vi "Main3.vi"() -> ()   [LabVIEW 2014]
doc: "The myRIO Project template acquires acceleration data from the onboard accelerometer and displays the changes of acceleration values in a waveform chart."
uses:
  C:/Program Files (x86)/National Instruments/LabVIEW 2014/examples/robotics/Vision/Color Tracking/HueSlider.ctl
  <vilib>/myRIO/Instrument Drivers/Onboard IO/AI/typedefs/AI Reference.ctl
  <vilib>/myRIO/Common/Instrument Driver Framework/Utilities/typedefs/myRIO Generic Hardware Reference.ctl
  <vilib>/myRIO/Common/Instrument Driver Framework/Utilities/typedefs/Hardware Version Enum.ctl
  <vilib>/myRIO/Common/Instrument Driver Framework/Utilities/typedefs/myRIO v1.0 Reference.ctl
  <vilib>/myRIO/Common/Instrument Driver Framework/Utilities/typedefs/Generic FPGA Reference.ctl
  <vilib>/myRIO/Common/Instrument Driver Framework/myRIO v1.0/AI/typedefs/AI Channels List.ctl
  <vilib>/myRIO/Common/Instrument Driver Framework/myRIO v1.0/AI/typedefs/AI Channels Enum.ctl
  <vilib>/myRIO/Common/Instrument Driver Framework/Utilities/typedefs/Analog Scaling Constants List.ctl
  <vilib>/myRIO/Common/Instrument Driver Framework/Utilities/typedefs/Analog Scaling Constants.ctl
  <vilib>/userdefined/High Color/nirio_resource_hc.ctl
  <vilib>/myRIO/Instrument Drivers/Onboard IO/PWM/typedefs/PWM Reference.ctl
  <vilib>/myRIO/Common/Instrument Driver Framework/myRIO v1.0/PWM/typedefs/PWM Channels Enum.ctl
  <vilib>/myRIO/Instrument Drivers/Onboard IO/PWM/typedefs/PWM Configuration.ctl
  <vilib>/myRIO/Common/Instrument Driver Framework/Utilities/vis/Is FPGA Ref Available.vi
  <vilib>/myRIO/Common/Instrument Driver Framework/myRIO v1.0/AI/vis/myRIO v1.1 Open AI.vi
  <vilib>/myRIO/Instrument Drivers/Onboard IO/AI/vis/Read.vi
  <vilib>/myRIO/Common/Instrument Driver Framework/myRIO v1.0/PWM/vis/myRIO v1.1 Open PWM.vi
  <vilib>/myRIO/Instrument Drivers/Onboard IO/PWM/vis/Set Duty Cycle and Frequency.vi
  <vilib>/myRIO/Common/Instrument Driver Framework/Utilities/vis/Validate Channels.vi
  <vilib>/myRIO/Common/Instrument Driver Framework/myRIO v1.0/AI/vis/myRIO v1.0 Reserve AI.vi
  <vilib>/myRIO/Common/Instrument Driver Framework/myRIO v1.0/PWM/vis/myRIO v1.0 Reserve PWM.vi
  <vilib>/myRIO/Common/Instrument Driver Framework/myRIO v1.0/AI/vis/myRIO v1.0 Build MUX Configuration AI.vi
  <vilib>/myRIO/Common/Instrument Driver Framework/myRIO v1.0/Resource Manager/vis/myRIO v1.0 Reserve Channel List.vi
  <vilib>/myRIO/Common/Instrument Driver Framework/myRIO v1.0/PWM/vis/myRIO v1.0 Build MUX Configuration PWM.vi
  <vilib>/myRIO/Common/Instrument Driver Framework/myRIO v1.0/Resource Manager/vis/myRIO v1.0 Reserve Channel.vi
  <vilib>/myRIO/Common/Instrument Driver Framework/myRIO v1.0/Resource Manager/vis/myRIO v1.0 Unreserve Channel.vi
  <vilib>/myRIO/Common/Instrument Driver Framework/myRIO v1.0/Resource Manager/vis/myRIO v1.0 Create Configuration List.vi
  <vilib>/myRIO/Common/Instrument Driver Framework/myRIO v1.0/Resource Manager/vis/myRIO v1.0 Build Mutex Name.vi
  <vilib>/Utility/VariantDataType/GetNumericInfo.vi
  <vilib>/Utility/error.llb/Error Cluster From Error Code.vi
  <vilib>/myRIO/Common/Instrument Driver Framework/myRIO v1.0/myRIO v1.1 Open.vi
  <vilib>/myRIO/Common/Instrument Driver Framework/myRIO v1.0/AI/vis/myRIO v1.0 Get Scaling Constants AI.vi
  <vilib>/myRIO/Common/Instrument Driver Framework/Utilities/vis/IO Manager.vi
  <vilib>/myRIO/Common/Instrument Driver Framework/Utilities/vis/Configuration Manager.vi
  <vilib>/myRIO/Common/Instrument Driver Framework/myRIO v1.0/myRIO v1.0 Close.vi
  <vilib>/myRIO/Common/Instrument Driver Framework/myRIO v1.0/AI/vis/myRIO v1.0 Read AI.vi
  <vilib>/myRIO/Common/Instrument Driver Framework/myRIO v1.0/Resource Manager/vis/myRIO v1.0 Configure IO.vi
  <vilib>/myRIO/Common/Instrument Driver Framework/myRIO v1.0/PWM/vis/myRIO v1.0 Write PWM.vi
  <vilib>/myRIO/Express VI/Onboard IO/AI/AI Express VI.xnode
  <vilib>/myRIO/Instrument Drivers/Onboard IO/AI/vis/myRIO AI Open.xnode
  <vilib>/myRIO/Express VI/Onboard IO/PWM/PWM Express VI.xnode
  <vilib>/myRIO/Instrument Drivers/Onboard IO/PWM/vis/myRIO PWM Open.xnode
  <vilib>/myRIO/Instrument Drivers/Onboard IO/PWM/PWM.lvlib
  <vilib>/vision/driver/NI_Vision_Acquisition_Software.lvlib
  <vilib>/vision/NI_Vision_Development_Module.lvlib
  <vilib>/myRIO/Instrument Drivers/Onboard IO/AI/AI.lvlib
panel:
  out "웨이브폼 차트":dbl(graph)
  out "Image 2":T1(plugin-control)
  in  "Hue range":T2={"Min"=232, "Max"=21} scale=0.0..255.0
  in  "Stop 2":bool
  out "Image":T1(plugin-control)
  in  "Camera Name":refnum<k21>="cam3" caption="IMAQdx Session"
  # "Control Motor"
  # "Read Encoder"
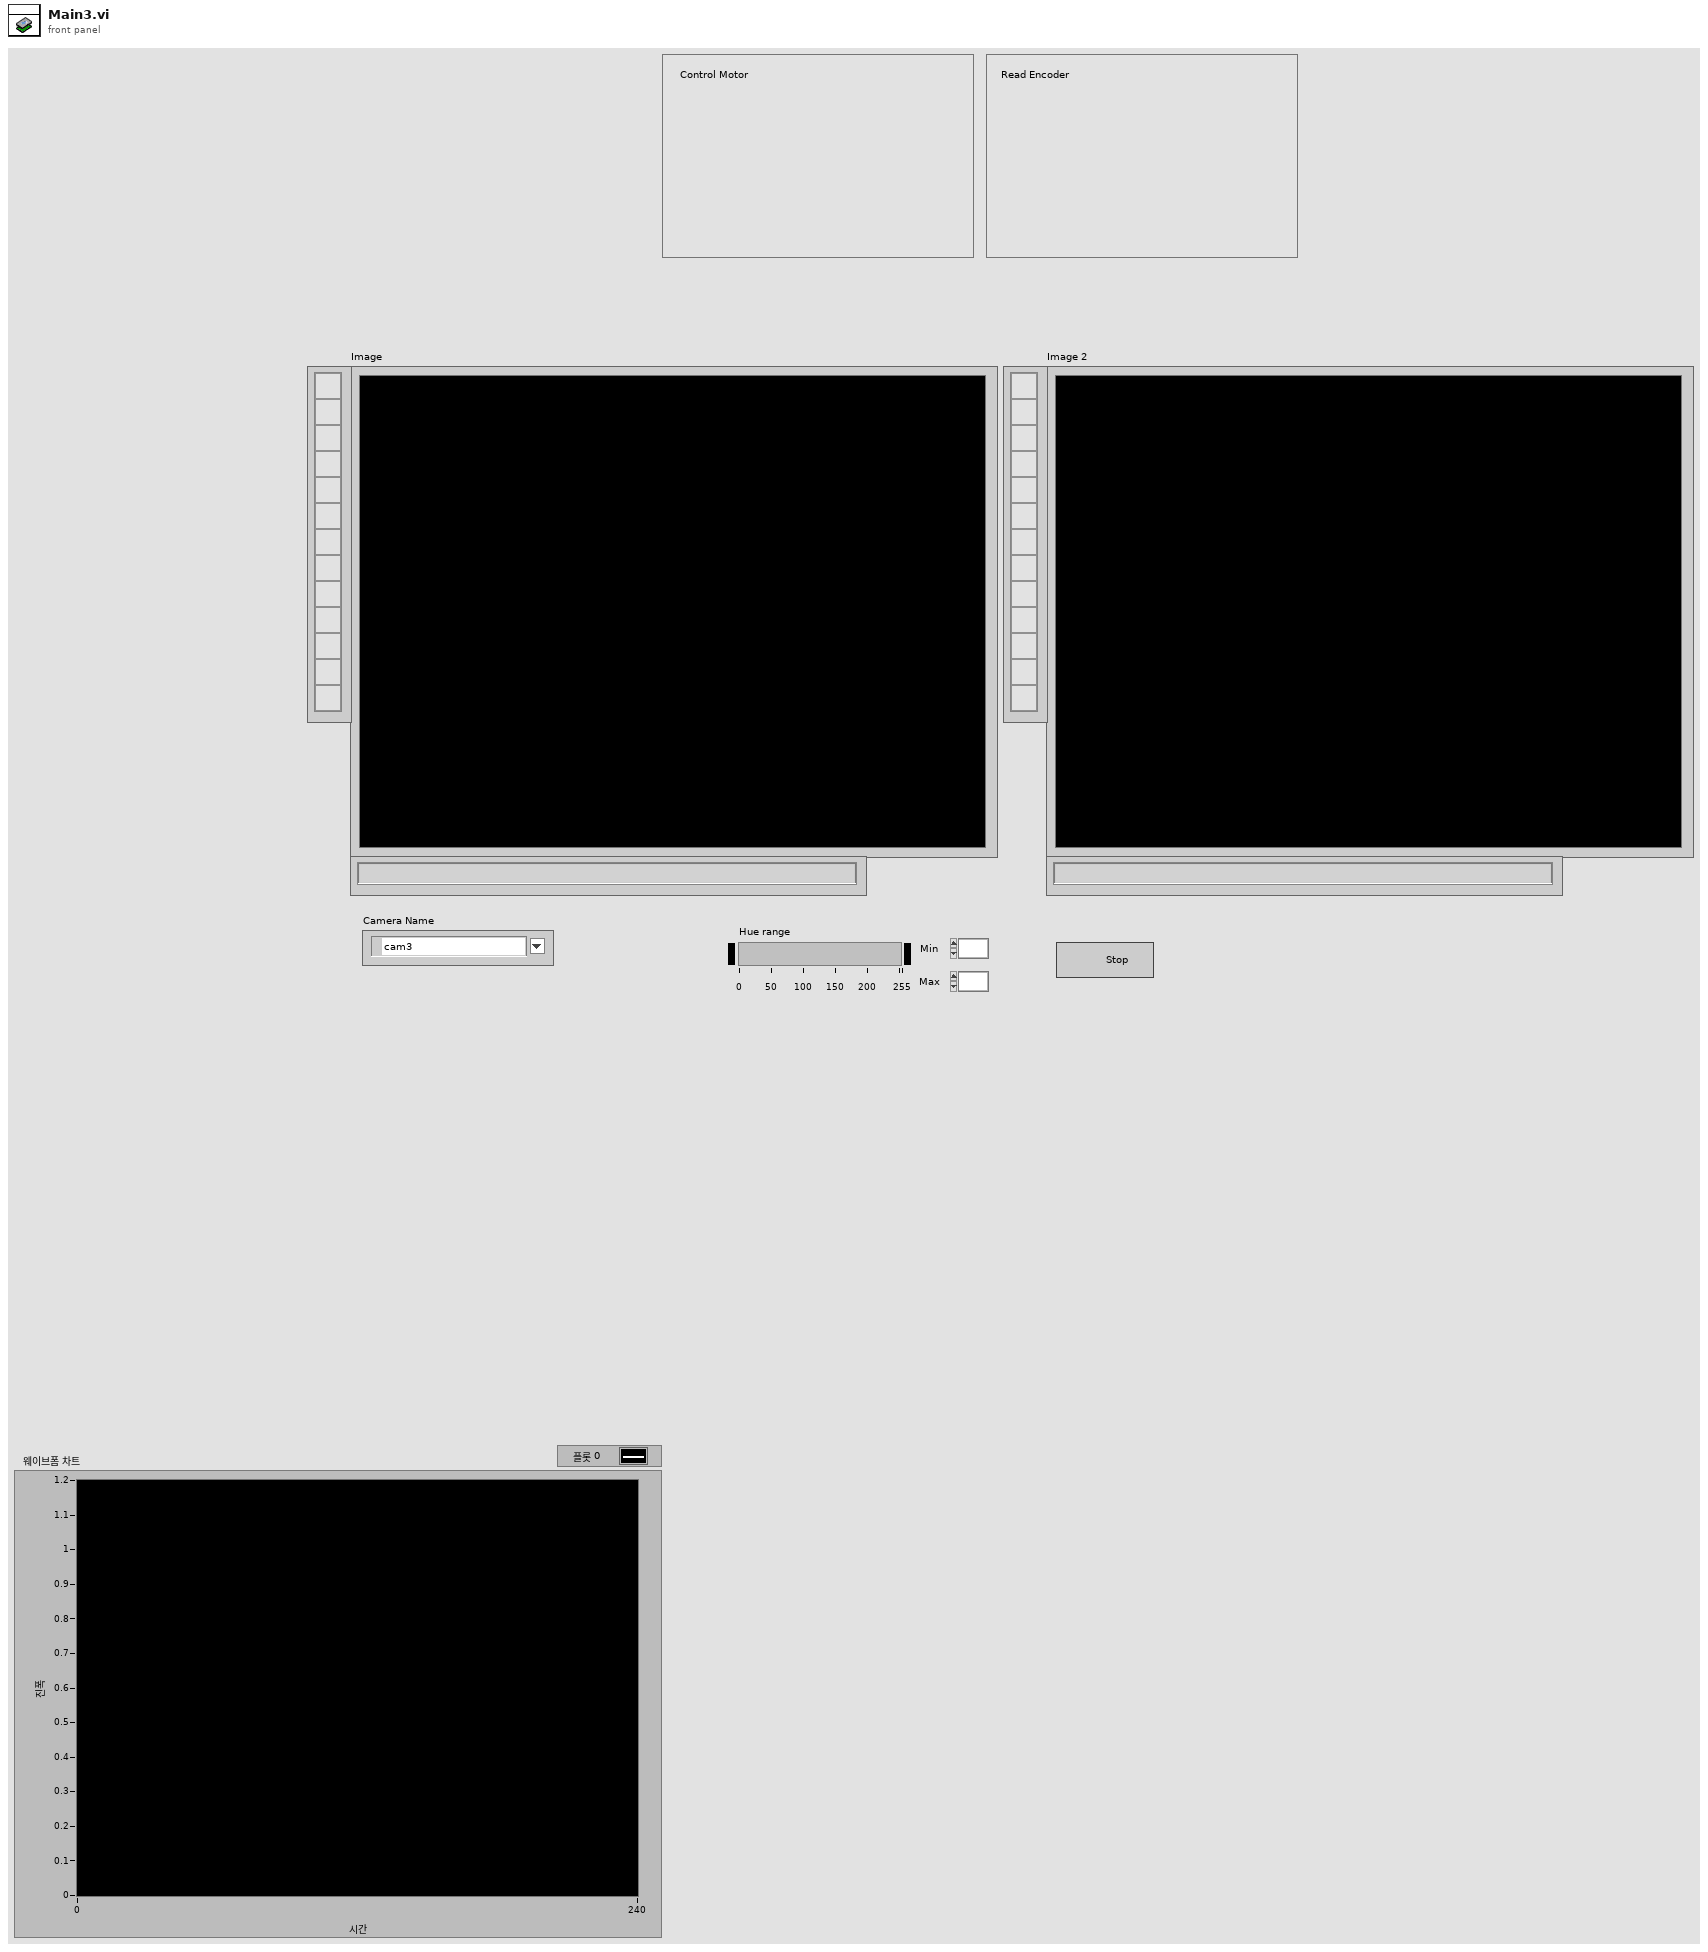
[diagram p1: front panel]
types:
  T1 = typedef "IMAQ Image.ctl" = refnum<image>
  T2 = typedef "HueSlider.ctl" = cluster{"Min":i32, "Max":i32}
  T3 = typedef "IMAQ Circle" = cluster{"Center X":i32, "Center Y":i32, "Inner Radius":i32, "Outer Radius":i32, "Start Angle":dbl, "End Angle":dbl}
  T4 = typedef "AI.lvlib/AI Reference.ctl" = cluster{"myRIO Reference":T5, "AI Channels List":T9, "AI Scaling Constants List":T11}
  T5 = typedef "myRIO Generic Hardware Reference.ctl" = cluster{"myRIO Model":T6, "myRIO Hardware Reference":T7}
  T6 = typedef "Hardware Version Enum.ctl" = enum16{"Unknown", "myRIO-1900", "myRIO-1950"}
  T7 = typedef "myRIO v1.0 Reference.ctl" = cluster{"Generic FPGA Reference":T8, "Allow multiple opens":bool}
  T8 = typedef "Generic FPGA Reference.ctl" = refnum<k20>
  T9 = typedef "AI Channels List.ctl" = T10[]
  T10 = typedef "AI Channels Enum.ctl" = enum16{"Not Connected", "AudioIn/Left", "AudioIn/Right", "C/AI0", "C/AI1", "A/AI0", "A/AI1", "A/AI2", "A/AI3", "B/AI0", "B/AI1", "B/AI2", "B/AI3"}
  T11 = typedef "Analog Scaling Constants List.ctl" = T12[]
  T12 = typedef "Analog Scaling Constants.ctl" = cluster{"LSB Weight (Volts)":dbl, "Offset (Volts)":dbl, "Signed?":bool}
  T13 = typedef "nirio_resource_hc.ctl" = tag
  T14 = typedef "IMAQ Rectangle" = cluster{"Left":i32, "Top":i32, "Right":i32, "Bottom":i32, "Rotation":dbl}
  T15 = typedef "PWM.lvlib/PWM Reference.ctl" = cluster{"myRIO Reference":T5, "PWM Channels Enum":T16, "PWM Configuration":T17}
  T16 = typedef "PWM Channels Enum.ctl" = enum16{"Not Connected", "C/PWM0", "C/PWM1", "A/PWM0", "A/PWM1", "A/PWM2", "B/PWM0", "B/PWM1", "B/PWM2"}
  T17 = typedef "PWM.lvlib/PWM Configuration.ctl" = cluster{"Frequency":dbl, "Duty Cycle":dbl}
  T18 = typedef "IMAQdx.ctl" = refnum<k21>
  T19 = cluster{"Global Rectangle":i32[], "Contours":cluster{"Contour Type":u32, "ROI Type":u32, "Points":i32[]}[]}
  T20 = cluster{"Center":cluster{"X":sgl, "Y":sgl}, "Radius":dbl}
  T21 = typedef "ROI Descriptor" = cluster{"Global Rectangle":i32[], "Contours":cluster{"ID":enum32{"External", "Internal"}, "Type":u32, "Coordinates":i32[]}[]}
  T22 = cluster{"Area":dbl, "Number of Holes":dbl, "Bounding Rect":cluster{"Left":dbl, "Top":dbl, "Right":dbl, "Bottom":dbl}, "Center of Mass":cluster{"X":dbl, "Y":dbl}, "Orientation":dbl, "Dimensions":cluster{"Width":dbl, "Height":dbl}}[]
  T23 = cluster{"Left":dbl, "Top":dbl, "Right":dbl, "Bottom":dbl}
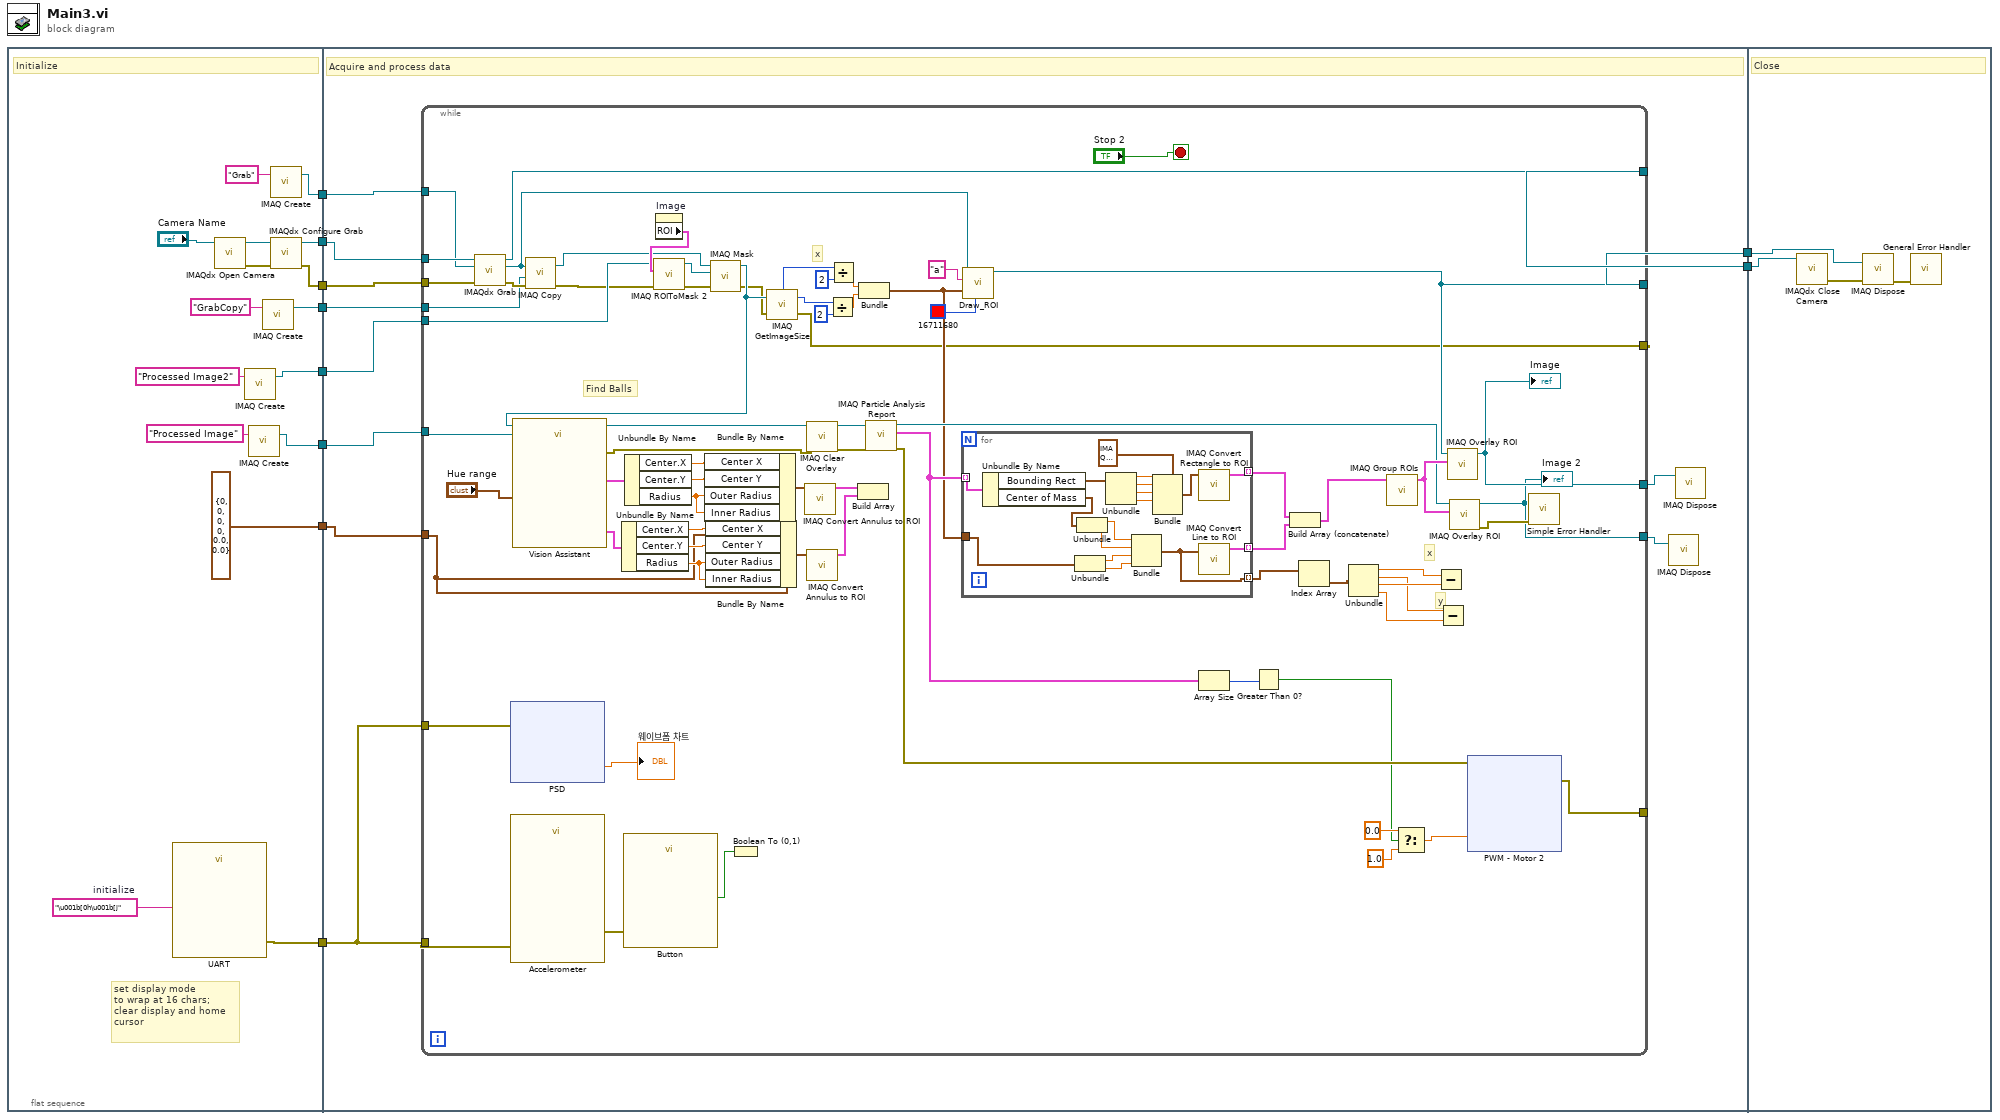
[diagram p0: block diagram]
diagram:
  n1 = flat-sequence {
    tunnel: [w22] -> w10
    tunnel: [w21] -> w9
    tunnel: [w20] -> w8
    tunnel: [T3 {"Center X"=0, "Center Y"=0, "Inner Radius"=0, "Outer Radius"=0, "Start Angle"=0.0, "End Angle"=0.0} ("Annulus")] -> w5
    tunnel: [w17] -> w4
    tunnel: [w15] -> w3
    tunnel: [w13] -> w2
    tunnel: [w12] -> w1
    tunnel: w10 -> [w38]
    tunnel: w9 -> [w37]
    tunnel: w8 -> [w36]
    tunnel: [w28] -> w7
    tunnel: [w35] -> w6
    tunnel: w5 -> [w34]
    tunnel: w4 -> [w33]
    tunnel: w3 -> [w30]
    tunnel: w2 -> [w29]
    tunnel: w1 -> [w27]
    tunnel: w7 -> [w202]
    tunnel: w6 -> [w201]
    frame #0 {
      w11 = "\u001b[0h\u001b[j"  # initialize
      # "set display mode\nto wrap at 16 chars;\nclear display and home\ncursor"
      # "Initialize"
      n2 = call "UART"("Characters to Write"=w11) -> ("error out"=w12:errorcluster)  [unwired: 25 in, 1 out]
      n3 = call <vilib>:"IMAQdx Open Camera.vi"("Session In"="Camera Name") -> ("error out"=w26:errorcluster, "Session Out"=w25:T18)  [unwired: 2 in, 7 out]
      n4 = call "IMAQ Create"("Image Name"="Processed Image2") -> ("New Image"=w15:T1)  [unwired: 3 in, 2 out]
      n5 = call "IMAQ Create"("Image Name"="Processed Image") -> ("New Image"=w17:T1)  [unwired: 3 in, 2 out]
      n6 = call "IMAQ Create"("Image Name"="GrabCopy") -> ("New Image"=w13:T1)  [unwired: 3 in, 2 out]
      n7 = call "IMAQ Create"("Image Name"="Grab") -> ("New Image"=w22:T1)  [unwired: 3 in, 2 out]
      n8 = call <vilib>:"IMAQdx Configure Grab.vi"("error in"=w26, "Session In"=w25) -> ("error out"=w20:errorcluster, "Session Out"=w21:T18)  [unwired: 8 out]
    }
    frame #1 {
      # "Acquire and process data"
      n9 = while {
        tunnel: [w108] -> w35
        tunnel: w36 -> [w110]
        tunnel: w37 -> [w111]
        tunnel: w38 -> [w109]
        tunnel: w34 -> [w90]
        tunnel: w33 -> [w89]
        tunnel: [w88] -> _
        tunnel: [w55] -> w32
        tunnel: [w54] -> w31
        tunnel: w30 -> [w78]
        tunnel: w29 -> [w63]
        tunnel: [w56] -> w28
        tunnel: [w52] -> _
        tunnel: w27 -> [w49]
        tunnel: w27 -> [w40]
        stop <- "Stop 2" stop-if-true
        # "y"
        # "x"
        # "x"
        # "Find Balls"
        n10 = call <vilib>:"IMAQdx Grab.vi"("error in"=w110, "Image In"=w109, "Session In"=w111) -> ("error out"=w65:errorcluster, "Image Out"=w61:T1, "Session Out"=w108:T18)  [unwired: 1 in, 5 out]
        n11 = xnode "PSD"("error in (no error)"=w40) -> ("C/AI0 (C/AI0 (AI0))"=→"웨이브폼 차트":dbl)  [unwired: 1 out]
        n12 = call "Accelerometer"("error in (no error)"=w49) -> ("error out"=w50:errorcluster)  [unwired: 23 in, 3 out]
        n13 = call "IMAQ Copy"("error in (no error)"=w65, "Image Dst"=w63, "Image Src"=w61) -> ("error out"=w64:errorcluster, "Image Dst Out"=w62:T1)  [unwired: 3 in]
        n14 = call "Button"("error in (no error)"=w50) -> ("Value"=w51:bool)  [unwired: 25 in, 1 out]
        n15 = property on="Image" class="ImageControl"() -> ("ROI"=w80:T19)  [unwired: 2 in, 2 out]
        n16 = call "IMAQ ROIToMask 2"("error in (no error)"=w64, "ROI Descriptor"=w80, "Image"=w78) -> ("error out"=w76:errorcluster, "Image Out"=w77:T1)  [unwired: 6 in, 1 out]
        n17 = call "IMAQ Mask"("error in (no error)"=w76, "Image Mask"=w77, "Image Src"=w62) -> ("error out"=w53:errorcluster, "Image Dst Out"=w60:T1)  [unwired: 2 in]
        n18 = call "Vision Assistant"("Image In"=w60, "Image Dst"=w89, "Red or Hue Range (Color Threshold)"="Hue range") -> ("Image Out"=w103:T1, "Best Circle (Fit Circle Ball 1)"=w91:T20, "Best Circle (Fit Circle Ball 2)"=w100:T20, "error out"=w105:errorcluster)  [unwired: 1 in, 20 out]
        n19 = Unbundle By Name(w100) -> ("Center.X"=w94:sgl, "Center.Y"=w95:sgl, "Radius"=w101:dbl)
        n20 = Unbundle By Name(w91) -> ("Center.X"=w92:sgl, "Center.Y"=w93:sgl, "Radius"=w102:dbl)
        n21 = Bundle By Name(cluster=w90, "Center X"=w92, "Center Y"=w93, "Outer Radius"=w102, "Inner Radius"=w102) -> (w96:T3)
        n22 = Bundle By Name(cluster=w90, "Center X"=w94, "Center Y"=w95, "Outer Radius"=w101, "Inner Radius"=w101) -> (w97:T3)
        n23 = Boolean To (0,1)(Boolean=w51) -> ()  [unwired: 1 out]
        n24 = call "IMAQ GetImageSize"("Image"=w60, "error in (no error)"=w53) -> ("Y Resolution"=w70:i32, "X Resolution"=w73:i32, "error out"=w52:errorcluster)  [unwired: 2 in]
        n25 = call "IMAQ Convert Annulus to ROI"("Annulus"=w96) -> ("ROI Descriptor"=w98:T21)  [unwired: 1 in, 8 out]
        n26 = call "IMAQ Clear Overlay"("error in (no error)"=w105, "Image"=w103) -> ("error out"=w74:errorcluster, "Image Out"=w83:T1)  [unwired: 1 in, 7 out]
        n27 = call "IMAQ Convert Annulus to ROI"("Annulus"=w97) -> ("ROI Descriptor"=w99:T21)  [unwired: 1 in, 8 out]
        n28 = Divide(x=w70, y=2) -> (x/y=w68:dbl)
        n29 = Divide(x=w73, y=2) -> (x/y=w69:dbl)
        n30 = Build Array(w98, w99) -> ()  [unwired: 1 out]
        n31 = Bundle(w69, w68) -> (w59:cluster{dbl, dbl})  [unwired: 1 in]
        n32 = call "IMAQ Particle Analysis Report"("error in (no error)"=w74, "Image"=w83) -> ("error out"=w81:errorcluster, "Particle Reports (Pixels)"=w75:T22, "Image Out (duplicate)"=w82:T1)  [unwired: 4 in, 3 out]
        n33 = for {
          tunnel: w75 -> [w165] mode=indexing
          tunnel: [w157] -> w58 mode=indexing
          tunnel: w59 -> [w153]
          tunnel: [w150] -> w48 mode=indexing
          tunnel: [w149] -> w47 mode=indexing
          n34 = Unbundle By Name(w165) -> ("Bounding Rect"=w163:T23, "Center of Mass"=w156:cluster{"X":dbl, "Y":dbl})
          n35 = Unbundle(w153) -> (w152:dbl, w151:dbl)
          n36 = Unbundle(w156) -> ("X"=w155:dbl, "Y"=w154:dbl)
          n37 = Unbundle(w163) -> ("Left"=w162:dbl, "Top"=w161:dbl, "Right"=w160:dbl, "Bottom"=w159:dbl)
          n38 = Bundle("X"=w155, "Y"=w154, w152, w151) -> (w149:cluster{"X":dbl, "Y":dbl, dbl, dbl})  [unwired: 1 in]
          n39 = Bundle(cluster=T14 {"Left"=0, "Top"=0, "Right"=0, "Bottom"=0, "Rotation"=0.0} ("Rectangle"), "Left"=w162, "Top"=w161, "Right"=w160, "Bottom"=w159) -> (w158:T14)  [unwired: 1 in]
          n40 = call "IMAQ Convert Rectangle to ROI"("Rectangle"=w158) -> ("ROI Descriptor"=w157:T21)  [unwired: 8 in, 1 out]
          n41 = call "IMAQ Convert Line to ROI"("Line"=w149) -> ("ROI Descriptor"=w150:T21)  [unwired: 8 in, 1 out]
        }
        n42 = call "Draw_ROI.vi"("Color"=u32 16711680, "클러스터"=w59, "Group"="a", "참조 번호 입력"=w61) -> ("참조 번호 출력"=w56:T1)  [unwired: 7 in]
        n43 = Array Size(array=w75) -> (size(s)=w87:i32)
        n44 = Greater Than 0?(x=w87) -> (x > 0?=w39:bool)
        n45 = Build Array (concatenate)(w58, w48) -> (w57:T21[])
        n46 = Index Array(array=w47) -> (element=w46:cluster{"X":dbl, "Y":dbl, dbl, dbl})  [unwired: 1 in]
        n47 = Unbundle(w46) -> ("X"=w45:dbl, "Y"=w43:dbl, w44:dbl, w42:dbl)
        n48 = call "IMAQ Group ROIs"("ROI Descriptors"=w57) -> ("ROI Descriptor out"=w104:T21)  [unwired: 1 in, 3 out]
        n49 = Select(t=0.0, s=w39, f=1.0) -> (s? t:f=w84:dbl)
        n50 = Subtract(x=w45, y=w44) -> ()  [unwired: 1 out]
        n51 = Subtract(x=w43, y=w42) -> ()  [unwired: 1 out]
        n52 = call "IMAQ Overlay ROI"("ROI Descriptor"=w104, "Image"=w56) -> ("Image Out"=w55:T1)  [unwired: 4 in, 5 out]
        "Image" <- w55
        n53 = call "IMAQ Overlay ROI"("ROI Descriptor"=w104, "Image"=w82) -> ("error out"=w106:errorcluster, "Image Out"=w54:T1)  [unwired: 4 in, 4 out]
        "Image 2" <- w54
        n54 = xnode "PWM - Motor 2"("Duty Cycle"=w84, "error in (no error)"=w81) -> ("error out"=w88:errorcluster)
        n55 = call <vilib>:"Simple Error Handler.vi"("error in (no error)"=w106) -> ()  [unwired: 1 in, 8 out]
      }
      n56 = call "IMAQ Dispose"("Image"=w31) -> ()  [unwired: 5 in, 1 out]
      n57 = call "IMAQ Dispose"("Image"=w32) -> ()  [unwired: 5 in, 1 out]
    }
    frame #2 {
      # "Close"
      n58 = call <vilib>:"IMAQdx Close Camera.vi"("Session In"=w201) -> ("error out"=w204:errorcluster)  [unwired: 1 in, 9 out]
      n59 = call "IMAQ Dispose"("Image"=w202, "error in (no error)"=w204) -> ("error out"=w203:errorcluster)  [unwired: 4 in]
      n60 = call <vilib>:"General Error Handler.vi"("error in (no error)"=w203) -> ()  [unwired: 2 in, 13 out]
    }
  }
